vi "Path Points.vi"(2 "Smooth Segments":dbl, 3 "Commands":T1(array[cluster])) -> (0 "Array 2":cluster{"X":dbl, "Y":dbl}[](array[cluster]), 1 "Array":cluster{"X":dbl, "Y":dbl}[][](array[cluster]))   [LabVIEW 2019]
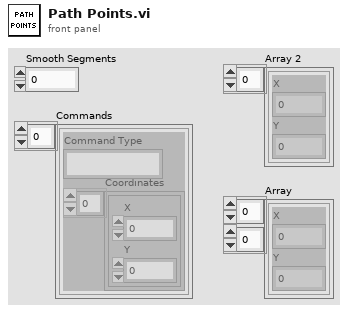
[diagram p1: front panel]
types:
  T1 = cluster{"Command Type":string, "Coordinates":cluster{"X":dbl, "Y":dbl}[]}[]
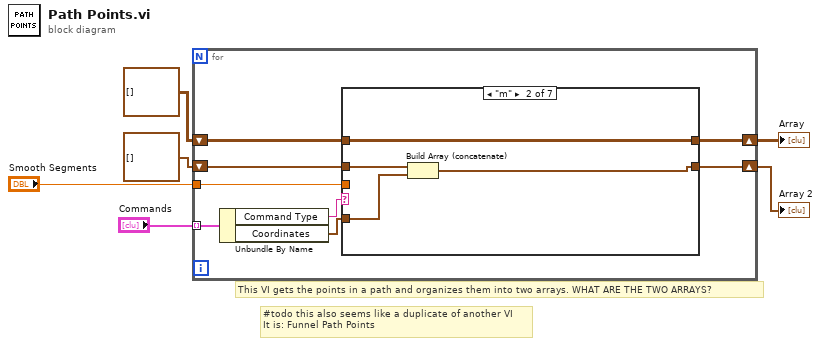
[diagram p0: block diagram]
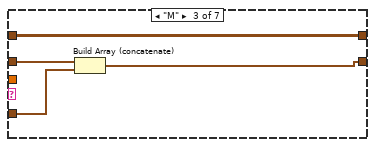
[diagram p3: hidden frame]
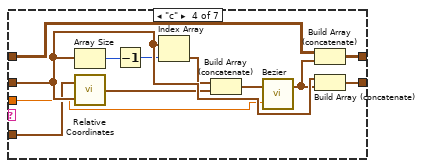
[diagram p4: hidden frame]
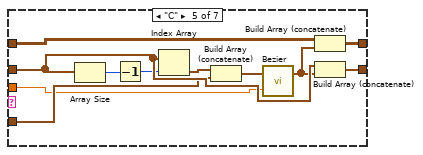
[diagram p5: hidden frame]
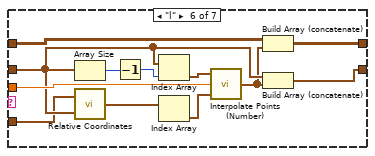
[diagram p6: hidden frame]
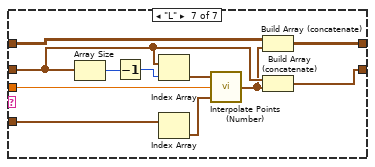
[diagram p7: hidden frame]
diagram:
  # "#todo this also seems like a duplicate of another VI\nIt is: Funnel Path Points"
  # "This VI gets the points in a path and organizes them into two arrays. WHAT ARE THE TWO ARRAYS?"
  n1 = for {
    tunnel: "Commands" -> [w7] mode=indexing
    shift-right: [w11] -> w5
    shift-left: cluster{"X":dbl, "Y":dbl}[] [] -> [w13]
    tunnel: "Smooth Segments" -> [w12]
    shift-right: [w9] -> w6
    shift-left: cluster{"X":dbl, "Y":dbl}[][] [] -> [w8]
    n2 = Unbundle By Name(w7) -> ("Command Type"=w14:string, "Coordinates"=w10:cluster{"X":dbl, "Y":dbl}[])
    n3 = case shown="\"m\"" w14 {
      tunnel: w10 -> [_ w18 w22 w28 w42 w51 w63]
      tunnel: w13 -> [w16 w19 w23 w36 w47 w52 w64]
      tunnel: [w16 w17 w21 w30 w43 w58 w69] -> w11
      tunnel: w12 -> [_ _ _ w29 w38 w59 w70]
      tunnel: [w15 w20 w24 w27 w40 w49 w62] -> w9
      tunnel: w8 -> [w15 w20 w24 w25 w39 w48 w60]
      frame "other letters", Default {
      }
      frame "m" {
        n4 = Build Array (concatenate)(w19, w18) -> (w17:cluster{"X":dbl, "Y":dbl}[])
      }
      frame "M" {
        n5 = Build Array (concatenate)(w23, w22) -> (w21:cluster{"X":dbl, "Y":dbl}[])
      }
      frame "c" {
        n6 = Array Size(array=w36) -> (size(s)=w32:i32)
        n7 = call "Relative Coordinates.vi"("All Coordinates"=w36, "Command Coordinates"=w28) -> ("Adjusted Command Coordinates"=w34:cluster{"X":dbl, "Y":dbl}[])
        n8 = Decrement(x=w32) -> (x-1=w31:i32)
        n9 = Index Array(array=w36, index=w31) -> (element=w35:cluster{"X":dbl, "Y":dbl})
        n10 = Build Array (concatenate)(w35, w34) -> (w33:cluster{"X":dbl, "Y":dbl}[])
        n11 = call "Bezier.vi"("Segments"=w29, "Parameters"=w33) -> ("Coordinate Array"=w26:cluster{"X":dbl, "Y":dbl}[])  [unwired: 1 out]
        n12 = Build Array (concatenate)(w25, w26) -> (w27:cluster{"X":dbl, "Y":dbl}[][])
        n13 = Build Array (concatenate)(w36, w26) -> (w30:cluster{"X":dbl, "Y":dbl}[])
      }
      frame "C" {
        n14 = Array Size(array=w47) -> (size(s)=w45:i32)
        n15 = Decrement(x=w45) -> (x-1=w44:i32)
        n16 = Index Array(array=w47, index=w44) -> (element=w46:cluster{"X":dbl, "Y":dbl})
        n17 = Build Array (concatenate)(w46, w42) -> (w37:cluster{"X":dbl, "Y":dbl}[])
        n18 = call "Bezier.vi"("Segments"=w38, "Parameters"=w37) -> ("Coordinate Array"=w41:cluster{"X":dbl, "Y":dbl}[])  [unwired: 1 out]
        n19 = Build Array (concatenate)(w39, w41) -> (w40:cluster{"X":dbl, "Y":dbl}[][])
        n20 = Build Array (concatenate)(w47, w41) -> (w43:cluster{"X":dbl, "Y":dbl}[])
      }
      frame "l" {
        n21 = Array Size(array=w52) -> (size(s)=w54:i32)
        n22 = call "Relative Coordinates.vi"("All Coordinates"=w52, "Command Coordinates"=w51) -> ("Adjusted Command Coordinates"=w57:cluster{"X":dbl, "Y":dbl}[])
        n23 = Decrement(x=w54) -> (x-1=w53:i32)
        n24 = Index Array(array=w52, index=w53) -> (element=w56:cluster{"X":dbl, "Y":dbl})
        n25 = Index Array(array=w57) -> (element=w55:cluster{"X":dbl, "Y":dbl})  [unwired: 1 in]
        n26 = call "Interpolate Points (Number).vi"("End Point"=w55, "Number of Points"=w59, "Start Point"=w56) -> ("Output Point Array"=w50:cluster{"X":dbl, "Y":dbl}[])
        n27 = Build Array (concatenate)(w48, w50) -> (w49:cluster{"X":dbl, "Y":dbl}[][])
        n28 = Build Array (concatenate)(w52, w50) -> (w58:cluster{"X":dbl, "Y":dbl}[])
      }
      frame "L" {
        n29 = Array Size(array=w64) -> (size(s)=w66:i32)
        n30 = Decrement(x=w66) -> (x-1=w65:i32)
        n31 = Index Array(array=w64, index=w65) -> (element=w68:cluster{"X":dbl, "Y":dbl})
        n32 = Index Array(array=w63) -> (element=w67:cluster{"X":dbl, "Y":dbl})  [unwired: 1 in]
        n33 = call "Interpolate Points (Number).vi"("End Point"=w67, "Number of Points"=w70, "Start Point"=w68) -> ("Output Point Array"=w61:cluster{"X":dbl, "Y":dbl}[])
        n34 = Build Array (concatenate)(w60, w61) -> (w62:cluster{"X":dbl, "Y":dbl}[][])
        n35 = Build Array (concatenate)(w64, w61) -> (w69:cluster{"X":dbl, "Y":dbl}[])
      }
    }
  }
  "Array" <- w6
  "Array 2" <- w5
